vi "Add Message Command.vi"(8 "error in (no error)":errorcluster, 11 "Message in":T1 format="%.0x") -> (0 "error out":errorcluster, 2 "Command Section Ptr":T1=18446744073709551615 format="%.0x", 3 "Message out":T1 format="%.0x")   [LabVIEW 2020, in "Instrument Addon Scripting API.lvlib"]
uses:
  Instrument Addon Scripting API.lvlib
  <vilib>/NI VeriStand/Custom Device API/Custom Device Item Ref.ctl
  Shared Directory/Constants.vi
  Shared Directory/Instrument Addon Shared.lvlib
  <vilib>/NI VeriStand/Custom Device API/Custom Device API.lvlib
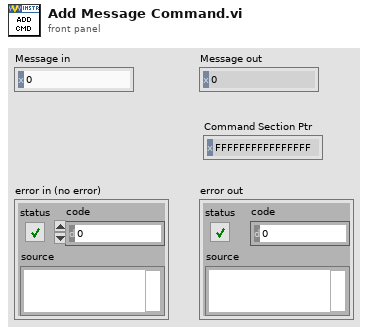
[diagram p1: front panel]
types:
  T1 = typedef "Custom Device API.lvlib/Custom Device Item Ref.ctl" = u64
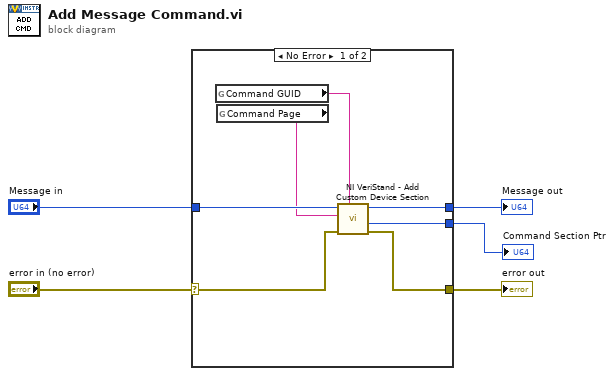
[diagram p0: block diagram]
diagram:
  n1 = case shown="No Error" "error in (no error)" {
    selector: "error in (no error)" -> [w7 w14]
    tunnel: "Message in" -> [w12 w13]
    tunnel: [w11 w13] -> w4
    tunnel: [w10 w14] -> w3
    tunnel: [w6 _] -> w1
    frame No Error {
      n2 = global read "Constants.vi" "Command GUID"() -> (w8:string)
      n3 = global read "Constants.vi" "Command Page"() -> (w9:string)
      n4 = call <vilib>:"NI VeriStand - Add Custom Device Section.vi"("GUID (Default Section)"=w8, "error in (no error)"=w7, "Section Name"=w9, "Parent Ref in"=w12) -> ("error out"=w10:errorcluster, "Section Ptr"=w6:T1, "Parent Ref out"=w11:T1)  [unwired: 4 in, 1 out]
    }
    frame Error {
    }
  }
  "Message out" <- w4
  "error out" <- w3
  "Command Section Ptr" <- w1
